vi "Log View for Energy Level (single value).vi"(2 "channel info":T1={"sensor sensitivity [mV/EU]"=1000.0, "engineering units"=1, "dB reference [EU]"=1.0, "custom label"="EU", "weighting filter"=0, "pregain [dB]"=0.0} {"pregain [dB]" format="%.2f"; "weighting filter" items=["Linear", "A-weighting", "B-weighting", "C-weighting", "ITU-R 468-4", "Dolby", "CCITT", "C-message"]; "dB reference [EU]" format="%^.1e"; "engineering units" items=["custom..."=0, "V"=1, "A"=21, "Pa"=2, "N"=20, "g"=3, "m/s^2"=4, "m/s"=5, "m"=6, "mm/s"=12, "mm"=13, "microns/s"=14, "microns"=15, "in/s^2"=7, "in/s"=8, "in"=9, "mils/s"=10, "mils"=11, "rad/s^2"=16, "rad/s"=17, "rad"=18, "strain"=19]; "sensor sensitivity [mV/EU]" format="%.2f"}, 3 "view mode":enum16{"Power", "Amplitude"}(ring), 4 "dB On (T)":bool=TRUE, 5 "energy level [EU^2 rms]":dbl format="%.2f") -> (0 "unit label":string, 1 "log view [dB EU]":dbl format="%.2f")   [LabVIEW 2017]
uses:
  <vilib>/addons/Sound and Vibration/compatibility/Controls/svl_Channel Info.ctl
  <vilib>/addons/Sound and Vibration/compatibility/Controls/svl_Engineering Units Text Ring.ctl
  <vilib>/addons/Sound and Vibration/compatibility/Controls/svl_Weighting Filter Text Ring.ctl
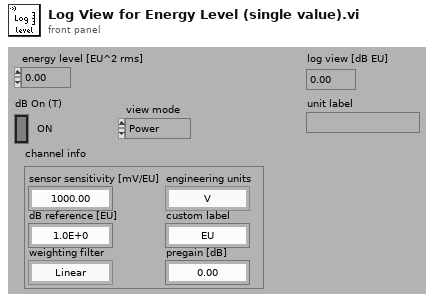
[diagram p1: front panel]
types:
  T1 = typedef "svl_Channel Info.ctl" = cluster{"sensor sensitivity [mV/EU]":dbl, "engineering units":T2, "dB reference [EU]":dbl, "custom label":string, "weighting filter":T3, "pregain [dB]":dbl}
  T2 = typedef "svl_Engineering Units Text Ring.ctl" = u16
  T3 = typedef "svl_Weighting Filter Text Ring.ctl" = u16
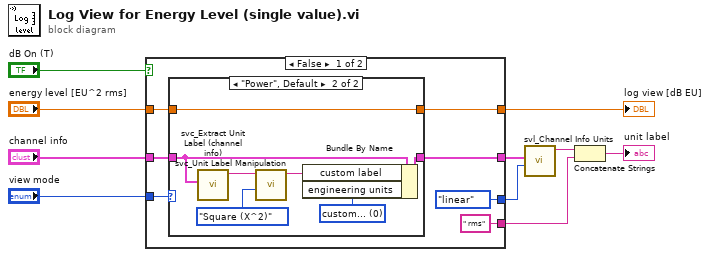
[diagram p0: block diagram]
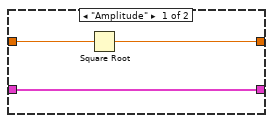
[diagram p2: hidden frame]
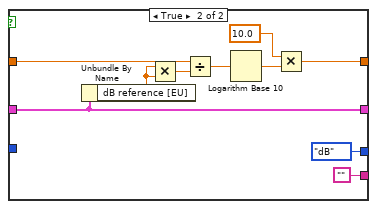
[diagram p3: hidden frame]
diagram:
  n1 = case shown="False" "dB On (T)" {
    tunnel: [w16 w37] -> w7
    tunnel: "channel info" -> [w12 w31]
    tunnel: "energy level [EU^2 rms]" -> [w15 w36]
    tunnel: "view mode" -> [w17 _]
    tunnel: [w11 w31] -> w3
    tunnel: [" rms" ""] -> w4
    tunnel: [enum16{"linear", "dB"}."linear" ("linear/dB") enum16{"linear", "dB"}."dB" ("linear/dB")] -> w1
    frame False {
      n2 = case shown="\"Power\", Default" w17 {
        tunnel: [w20 w26] -> w16
        tunnel: w15 -> [w19 w26]
        tunnel: w12 -> [w18 w24]
        tunnel: [w18 w23] -> w11
        frame "Amplitude" {
          n3 = Square Root(x=w19) -> (sqrt(x)=w20:dbl)
        }
        frame "Power", Default {
          w21 = u16 0 items=["custom...", "V", "Pa", "g", "m/s^2", "m/s", "m", "in/s^2", "in/s", "in", "mm", "mils", "A"] ("engineering units")
          n4 = call <vilib>:"svc_Extract Unit Label (channel info).vi"("channel info"=w24) -> ("unit label"=w25:string)  [unwired: 8 in, 2 out]
          n5 = call <vilib>:"svc_Unit Label Manipulation.vi"("operation"=enum16{"Square (X^2)", "Divide (X/Y)"}."Square (X^2)", "X unit label"=w25) -> ("resulting unit label"=w22:string)  [unwired: 5 in]
          n6 = Bundle By Name(cluster=w24, "custom label"=w22, "engineering units"=w21) -> (w23:T1)
        }
      }
    }
    frame True {
      n7 = Unbundle By Name(w31) -> ("dB reference [EU]"=w28:dbl)
      n8 = Multiply(x=w28, y=w28) -> (x*y=w34:dbl)
      n9 = Divide(x=w36, y=w34) -> (x/y=w35:dbl)
      n10 = Logarithm Base 10(1:w35) -> (0:w32:dbl)
      n11 = Multiply(x=10.0 ("y"), y=w32) -> (x*y=w37:dbl)
    }
  }
  "log view [dB EU]" <- w7
  n12 = call <vilib>:"svl_Channel Info Units.vi"("linear/dB"=w1, "channel info"=w3) -> ("unit label"=w2:string)  [unwired: 8 in, 1 out]
  n13 = Concatenate Strings(w2, w4) -> (→"unit label":string)
